vi "关键参数区.vi"(11 "数组":u16[](array[numeric]) format="%04xH") -> (3 "关键参数区":T1)   [LabVIEW 2016, in "斯坦道总磷总氮.lvlib"]
panel:
  # "共占用56 WORD"
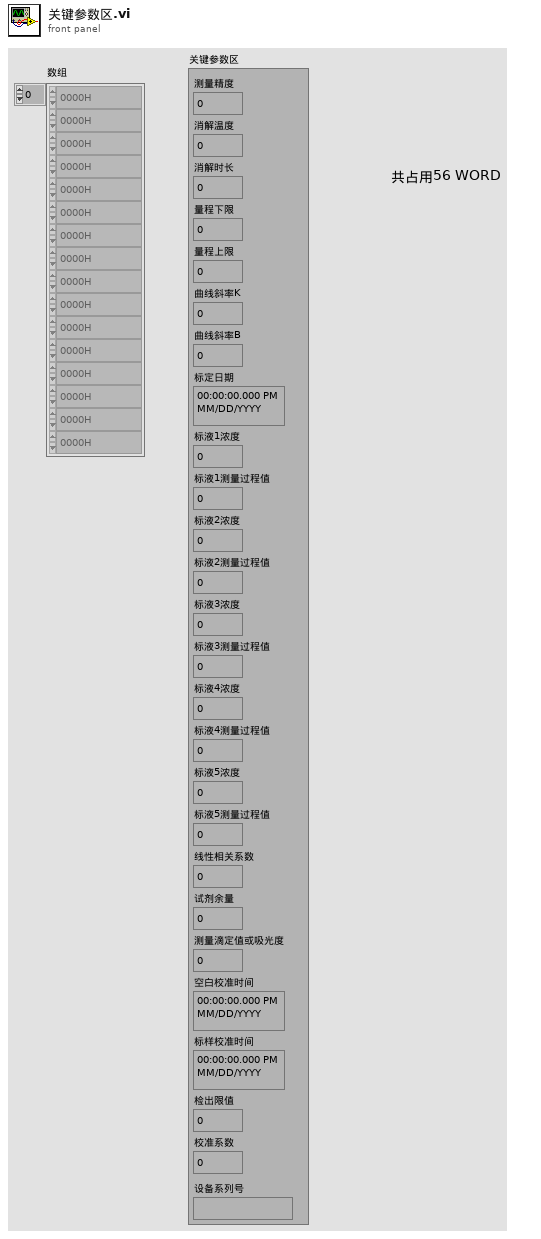
[diagram p1: front panel]
types:
  T1 = cluster{"测量精度":u16, "消解温度":u16, "消解时长":u16, "量程下限":sgl, "量程上限":sgl, "曲线斜率K":sgl, "曲线斜率B":sgl, "标定日期":timestamp, "标液1浓度":sgl, "标液1测量过程值":sgl, "标液2浓度":sgl, "标液2测量过程值":sgl, "标液3浓度":sgl, "标液3测量过程值":sgl, "标液4浓度":sgl, "标液4测量过程值":sgl, "标液5浓度":sgl, "标液5测量过程值":sgl, "线性相关系数":sgl, "试剂余量":u32, "测量滴定值或吸光度":sgl, "空白校准时间":timestamp, "标样校准时间":timestamp, "检出限值":sgl, "校准系数":sgl, "设备系列号":string}
  T2 = cluster{"WORD":u16, "WORD":u16, "WORD":u16, "FLOAT":sgl, "FLOAT":sgl, "FLOAT":sgl, "FLOAT":sgl, "time stamp":timestamp, "FLOAT":sgl, "FLOAT":sgl, "FLOAT":sgl, "FLOAT":sgl, "FLOAT":sgl, "FLOAT":sgl, "FLOAT":sgl, "FLOAT":sgl, "FLOAT":sgl, "FLOAT":sgl, "FLOAT":sgl, "DWORD":i32, "FLOAT":sgl, "time stamp":timestamp, "time stamp":timestamp, "FLOAT":sgl, "FLOAT":sgl, "string":string}
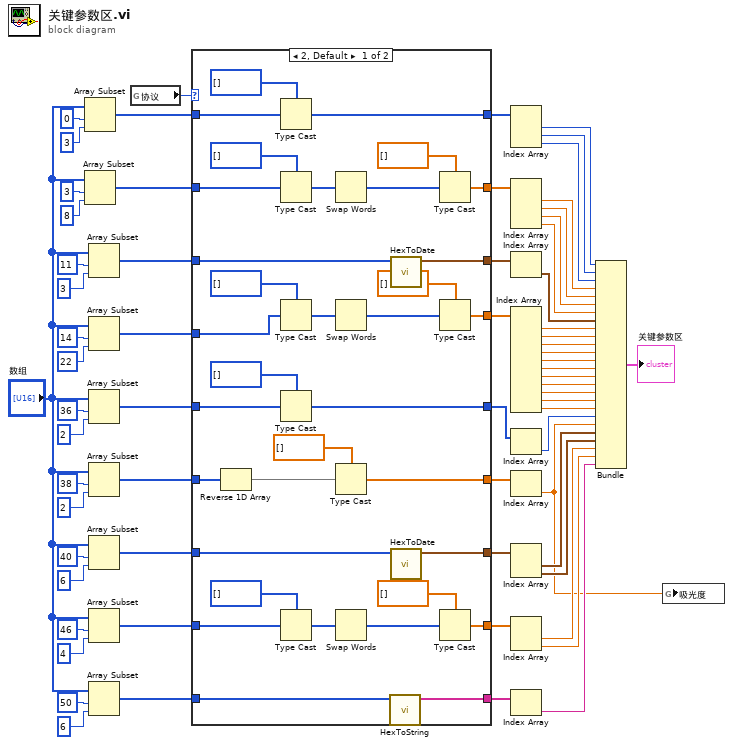
[diagram p0: block diagram]
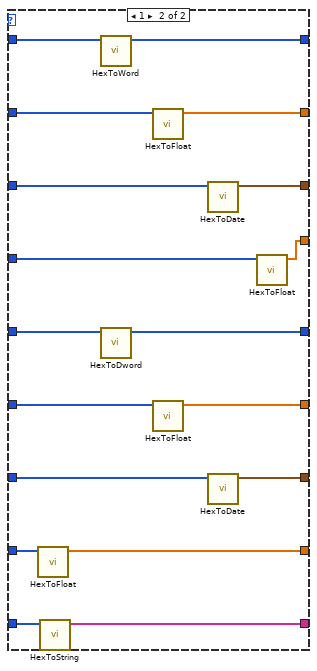
[diagram p2: hidden frame]
diagram:
  n1 = Array Subset(array="数组", index=0 ("索引"), length=3 ("长度")) -> (w60:u16[])
  n2 = Array Subset(array="数组", index=3 ("索引"), length=8 ("长度")) -> (w56:u16[])
  n3 = Array Subset(array="数组", index=11 ("索引"), length=3 ("长度")) -> (w48:u16[])
  n4 = Array Subset(array="数组", index=14 ("索引"), length=22 ("长度")) -> (w43:u16[])
  n5 = Array Subset(array="数组", index=36 ("索引"), length=2 ("长度")) -> (w18:u16[])
  n6 = Array Subset(array="数组", index=38 ("索引"), length=2 ("长度")) -> (w19:u16[])
  n7 = Array Subset(array="数组", index=40 ("索引"), length=6 ("长度")) -> (w31:u16[])
  n8 = Array Subset(array="数组", index=46 ("索引"), length=4 ("长度")) -> (w26:u16[])
  n9 = Array Subset(array="数组", index=50 ("索引"), length=6 ("长度")) -> (w20:u16[])
  n10 = global read "总磷总氮断电保存全局变量.vi" "协议"() -> (w2:u16)
  n11 = case shown="2, Default" w2 {
    tunnel: w60 -> [w83 w117]
    tunnel: [w82 w116] -> w59
    tunnel: w56 -> [w81 w115]
    tunnel: [w80 w114] -> w55
    tunnel: w48 -> [w79 w113]
    tunnel: [w78 w112] -> w47
    tunnel: w43 -> [w77 w111]
    tunnel: [w76 w110] -> w42
    tunnel: [w74 w109] -> w37
    tunnel: w31 -> [w71 w108]
    tunnel: [w70 w107] -> w30
    tunnel: w26 -> [w69 w106]
    tunnel: [w68 w105] -> w24
    tunnel: w20 -> [w67 w104]
    tunnel: w19 -> [w73 w103]
    tunnel: w18 -> [w75 w102]
    tunnel: [w72 w101] -> w14
    tunnel: [w66 w100] -> w4
    frame 2, Default {
      n12 = Reverse 1D Array(array=w73) -> (reversed array=w89:u16[])
      n13 = Type Cast(type=u16[] [], x=w83) -> (*(type *) &x=w82:u16[])
      n14 = Type Cast(type=i32[] [], x=w81) -> (*(type *) &x=w97:i32[])
      n15 = Type Cast(type=i32[] [], x=w77) -> (*(type *) &x=w93:i32[])
      n16 = Type Cast(type=u16[] [], x=w75) -> (*(type *) &x=w74:u16[])
      n17 = Type Cast(type=i32[] [], x=w69) -> (*(type *) &x=w85:i32[])
      n18 = Swap Words(1:w97) -> (0:w95:i32[])
      n19 = Swap Words(1:w93) -> (0:w91:i32[])
      n20 = Type Cast(type=sgl[] [], x=w89) -> (*(type *) &x=w72:sgl[])
      n21 = Swap Words(1:w85) -> (0:w87:i32[])
      n22 = call "HexToString.vi"("数组"=w67) -> ("STRING"=w66:string[])  [unwired: 10 in]
      n23 = call "HexToDate.vi"("数组"=w79) -> ("DATE"=w78:timestamp[])  [unwired: 10 in]
      n24 = call "HexToDate.vi"("数组"=w71) -> ("DATE"=w70:timestamp[])  [unwired: 10 in]
      n25 = Type Cast(type=sgl[] [], x=w95) -> (*(type *) &x=w80:sgl[])
      n26 = Type Cast(type=sgl[] [], x=w91) -> (*(type *) &x=w76:sgl[])
      n27 = Type Cast(type=sgl[] [], x=w87) -> (*(type *) &x=w68:sgl[])
    }
    frame 1 {
      n28 = call "HexToFloat.vi"("数组"=w106) -> ("FLOAT"=w105:sgl[])  [unwired: 10 in]
      n29 = call "HexToString.vi"("数组"=w104) -> ("STRING"=w100:string[])  [unwired: 10 in]
      n30 = call "HexToWord.vi"("数组"=w117) -> ("WORD"=w116:u16[])  [unwired: 10 in]
      n31 = call "HexToDword.vi"("数组"=w102) -> ("DWORD"=w109:i32[])  [unwired: 10 in]
      n32 = call "HexToFloat.vi"("数组"=w115) -> ("FLOAT"=w114:sgl[])  [unwired: 10 in]
      n33 = call "HexToFloat.vi"("数组"=w103) -> ("FLOAT"=w101:sgl[])  [unwired: 10 in]
      n34 = call "HexToDate.vi"("数组"=w113) -> ("DATE"=w112:timestamp[])  [unwired: 10 in]
      n35 = call "HexToDate.vi"("数组"=w108) -> ("DATE"=w107:timestamp[])  [unwired: 10 in]
      n36 = call "HexToFloat.vi"("数组"=w111) -> ("FLOAT"=w110:sgl[])  [unwired: 10 in]
    }
  }
  n37 = Index Array(array=w59) -> (element #1=w63:u16, element #2=w62:u16, element #3=w61:u16)  [unwired: 3 in]
  n38 = Index Array(array=w55) -> (element #1=w54:sgl, element #2=w53:sgl, element #3=w52:sgl, element #4=w51:sgl)  [unwired: 4 in]
  n39 = Index Array(array=w47) -> (element=w46:timestamp)  [unwired: 1 in]
  n40 = Index Array(array=w42) -> (element #1=w41:sgl, element #2=w40:sgl, element #3=w39:sgl, element #4=w38:sgl, element #5=w12:sgl, element #6=w11:sgl, element #7=w10:sgl, element #8=w9:sgl, element #9=w8:sgl, element #10=w7:sgl, element #11=w6:sgl)  [unwired: 11 in]
  n41 = Index Array(array=w37) -> (element=w34:i32)  [unwired: 1 in]
  n42 = Index Array(array=w14) -> (element=w1:sgl)  [unwired: 1 in]
  n43 = Index Array(array=w30) -> (element #1=w29:timestamp, element #2=w28:timestamp)  [unwired: 2 in]
  n44 = Index Array(array=w24) -> (element #1=w23:sgl, element #2=w13:sgl)  [unwired: 2 in]
  n45 = Index Array(array=w4) -> (element=w3:string)  [unwired: 1 in]
  n46 = Bundle("WORD"=w63, "WORD"=w62, "WORD"=w61, "FLOAT"=w54, "FLOAT"=w53, "FLOAT"=w52, "FLOAT"=w51, "time stamp"=w46, "FLOAT"=w41, "FLOAT"=w40, "FLOAT"=w39, "FLOAT"=w38, "FLOAT"=w12, "FLOAT"=w11, "FLOAT"=w10, "FLOAT"=w9, "FLOAT"=w8, "FLOAT"=w7, "FLOAT"=w6, "DWORD"=w34, "FLOAT"=w1, "time stamp"=w29, "time stamp"=w28, "FLOAT"=w23, "FLOAT"=w13, "string"=w3) -> (→"关键参数区":T2)  [unwired: 1 in]
  n47 = global write "总磷总氮断电保存全局变量.vi" "吸光度"(w1) -> ()
